vi "SysExe._Test Bat File Return Info.vi"() -> ()   [LabVIEW 2018]
panel:
  out "error out":errorcluster
  out "Rtn":i32
  out "StdErr":string
  out "StdOut":string
  in  "File":path
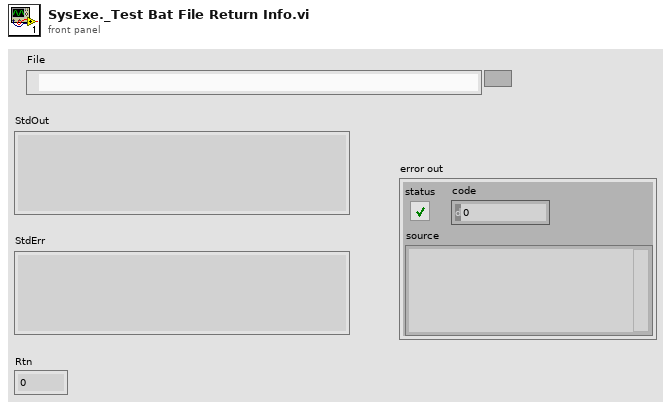
[diagram p1: front panel]
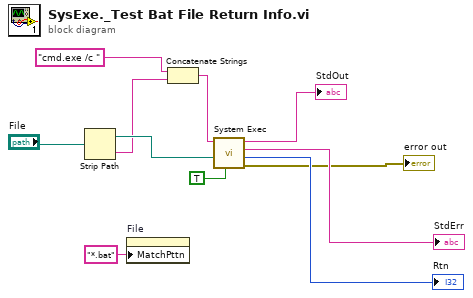
[diagram p0: block diagram]
diagram:
  n1 = Strip Path(path="File") -> (stripped path=w6:path, name=w4:string)
  n2 = property on="File" class="Path"("MatchPttn"="*.bat" ("Browse Options:Match Pattern")) -> ()  [unwired: 2 in, 2 out]
  n3 = Concatenate Strings("cmd.exe /c ", w4) -> (w3:string)
  n4 = call <vilib>:"System Exec.vi"("run minimized? (F)"=TRUE, "working directory"=w6, "command line"=w3) -> ("error out"=→"error out":errorcluster, "return code"=→"Rtn":i32, "standard error"=→"StdErr":string, "standard output"=→"StdOut":string)  [unwired: 5 in]
